vi "Delimiter Read 1.vi"(4 "error in (no error)":errorcluster, 6 "Container State":T3, 7 "Display State In":T2) -> (0 "error out":errorcluster, 2 "Value":T1, 3 "Display State Out":T2)   [LabVIEW 2012, in "Intellisense Xcontrol.xctl"]
uses:
  Intellisense Xcontrol.xctl
  <vilib>/_xctls/Container State.ctl
  State 1.ctl
  Delimiter Enum.ctl
  <vilib>/_xctls/XControlSupport.lvlib
panel:
  # "Replace the Value Indicator below with an Indicator of desired type.\nDo not remove this Indicator or the others from the connector pane. \nDo not change the connector pane pattern.\nThe Value Indicator should always be the second terminal from top on the output side in the connector pane."
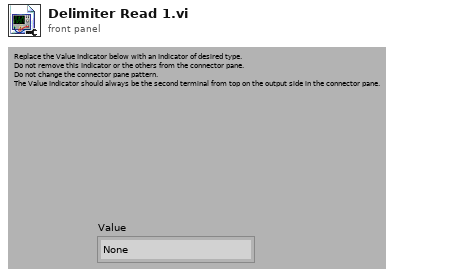
[diagram p1: front panel]
types:
  T1 = typedef "Intellisense Xcontrol.xctl/Delimiter Enum.ctl" = enum16{"None", "Space", "Dash \"-\"", "Slash \"/\"", "Backslash \"\\\"", "Colon", "Period", "Comma", "Line Feed"}
  T2 = typedef "Intellisense Xcontrol.xctl/State 1.ctl" = cluster{"Keyword Array":string[], "Auto-Complete On/Off":bool, "Delimiter":string}
  T3 = typedef "XControlSupport.lvlib/Container State.ctl" = cluster{"Indicator?":bool, "Run Mode?":bool, " Refnum":refnum<vi>}
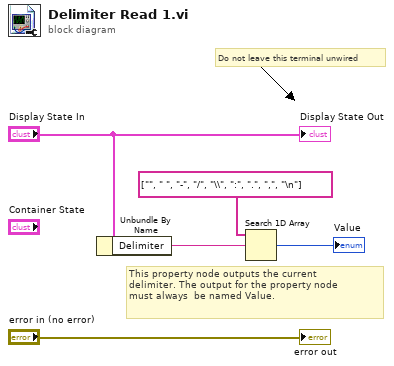
[diagram p0: block diagram]
diagram:
  # "This property node outputs the current\ndelimiter. The output for the property node\nmust always  be named Value."
  # "Do not leave this terminal unwired"
  n1 = Unbundle By Name("Display State In") -> ("Delimiter"=w3:string)
  n2 = Search 1D Array(1D array=string[] ["", " ", "-", "/", "\\", ":", ".", ",", "\n"], element=w3) -> (index of element=→"Value":i32)  [unwired: 1 in]
  "error out" <- "error in (no error)"
  "Display State Out" <- "Display State In"
